vi "SetData.vi"(5 "列":i32, 7 "行":i32, 8 "error":errorcluster caption="错误输入（无错误）", 10 "data":variant, 11 "Excel._Worksheet":refnum<k7>) -> (0 "error out":errorcluster caption="错误输出", 3 "Excel._Worksheet":refnum<k7>)   [LabVIEW 2014]
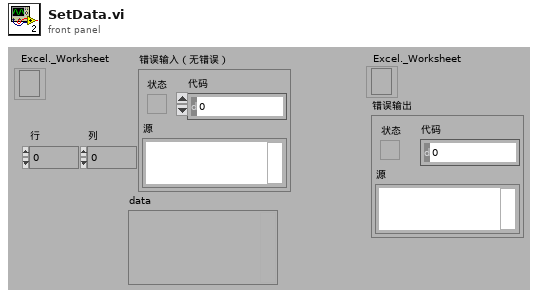
[diagram p1: front panel]
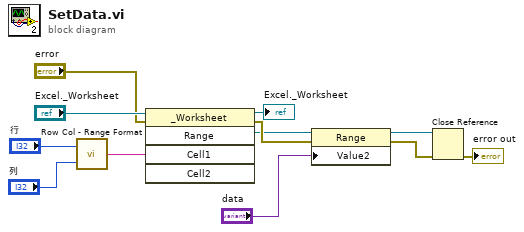
[diagram p0: block diagram]
diagram:
  n1 = call "Row Col - Range Format.vi"("Column"="列", "Row"="行") -> ("Output String"=w11:string)
  n2 = invoke class="_Worksheet" method="Range"(reference="Excel._Worksheet", error in="error", "Cell1"=w11) -> (reference out=→"Excel._Worksheet":refnum<k7>, error out=w5:errorcluster, "Range"=w1:refnum<k7>)  [unwired: 2 in, 2 out]
  n3 = property class="Range"(reference=w1, error in=w5, "Value2"="data") -> (reference out=w7:refnum<k7>, error out=w6:errorcluster)
  n4 = Close Reference(reference=w7, error in (no error)=w6) -> (error out=→"error out":errorcluster)
